vi "main.vi"() -> ()   [LabVIEW 2020]
uses:
  Controls/Estados.ctl
panel:
  out "Key":dbl
  in  "Keyboard":bool[][](array[boolean])
  in  "stop":bool
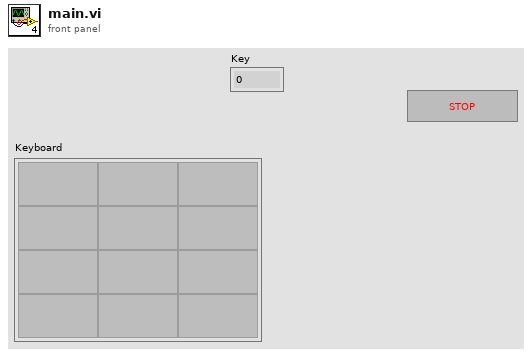
[diagram p1: front panel]
types:
  T1 = typedef "Estados.ctl" = enum16{"Init", "Scan", "Tone"}
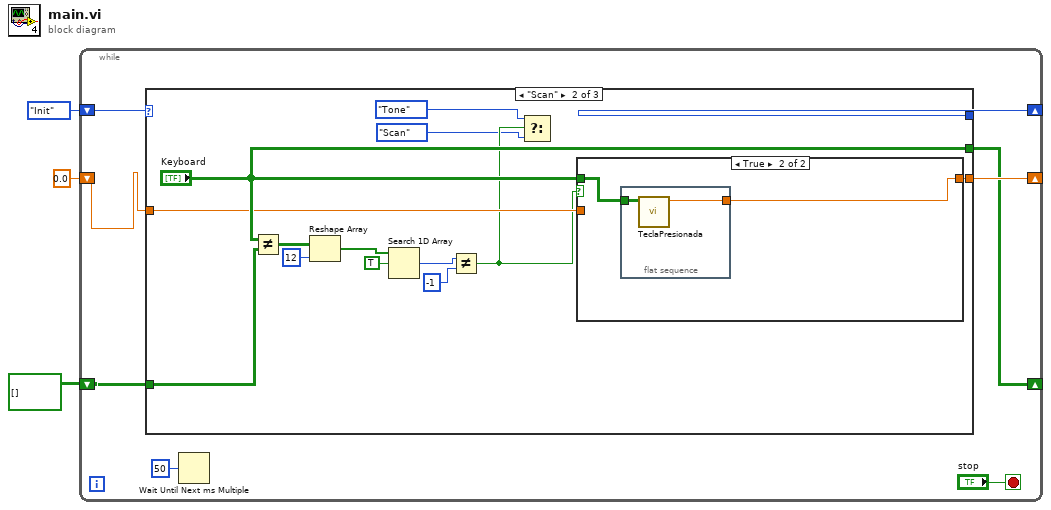
[diagram p0: block diagram]
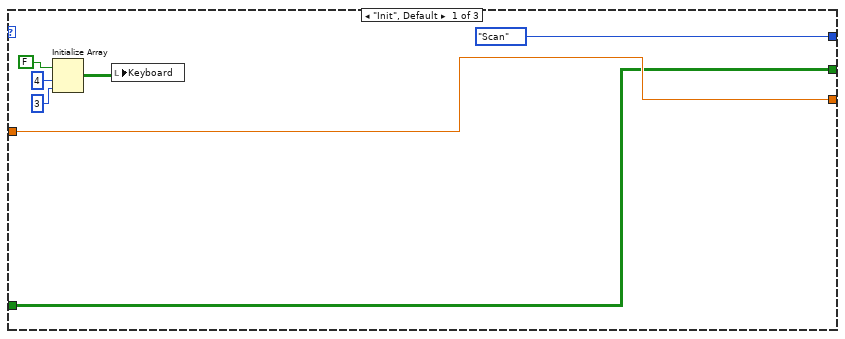
[diagram p2: hidden frame]
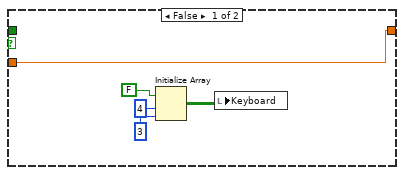
[diagram p3: hidden frame]
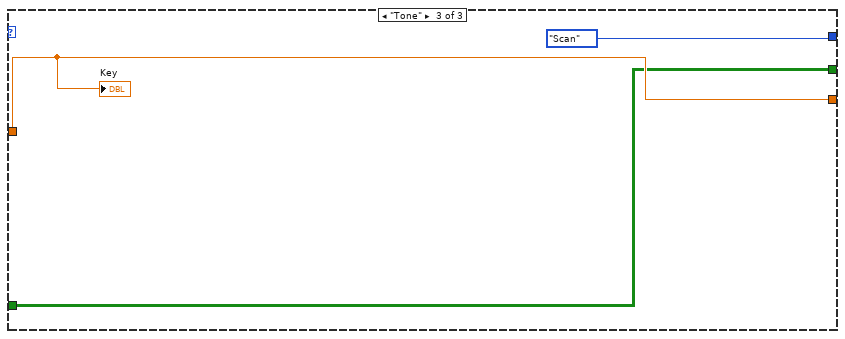
[diagram p4: hidden frame]
diagram:
  n1 = while {
    shift-right: [w8] -> _
    shift-left: Estados."Init" ("Estados") -> [w9]
    shift-right: [w7] -> _
    shift-left: 0.0 ("Numeric") -> [w6]
    shift-right: [w5] -> _
    shift-left: bool[][] [] ("Keyboard") -> [w4]
    stop <- "stop" stop-if-true
    n2 = case shown="\"Scan\"" w9 {
      tunnel: [Estados."Scan" ("Estados") _ Estados."Scan" ("Estados")] -> w8
      tunnel: [w13 w31 w43] -> w7
      tunnel: w6 -> [w13 w22 w43]
      tunnel: [w12 "Keyboard" w41] -> w5
      tunnel: w4 -> [w12 w29 w41]
      frame "Init", Default {
        n3 = Initialize Array(FALSE, 4 ("dimension size"), 3 ("dimension size")) -> (w14:bool[][])
        n4 = local write "Keyboard"(w14) -> ()
      }
      frame "Scan" {
        n5 = Not Equal?(x="Keyboard", y=w29) -> (x != y?=w28:bool[][])
        n6 = Reshape Array(w28, 12 ("dimension size")) -> (w26:bool[])
        n7 = Search 1D Array(1D array=w26, element=TRUE) -> (index of element=w24:i32)  [unwired: 1 in]
        n8 = Not Equal?(x=w24, y=-1) -> (x != y?=w21:bool)
        n9 = Select(t=Estados."Tone" ("Estados"), s=w21, f=Estados."Scan" ("Estados")) -> ()  [unwired: 1 out]
        n10 = case shown="True" w21 {
          tunnel: [w36 w38] -> w31
          tunnel: "Keyboard" -> [_ w37]
          tunnel: w22 -> [w36 _]
          frame False {
            n11 = Initialize Array(FALSE, 4 ("dimension size"), 3 ("dimension size")) -> (w35:bool[][])
            n12 = local write "Keyboard"(w35) -> ()
          }
          frame True {
            n13 = flat-sequence {
              tunnel: w37 -> [w39]
              tunnel: [w40] -> w38
              frame #0 {
                n14 = call "TeclaPresionada.vi"("Keyboard"=w39) -> ("Numeric"=w40:dbl)  [unwired: 10 in]
              }
            }
          }
        }
      }
      frame "Tone" {
        "Key" <- w43
      }
    }
    n15 = Wait Until Next ms Multiple(millisecond multiple=u32 50) -> ()  [unwired: 1 out]
  }
